vi "Updater Install Spartan Service.vi"(8 "error in (no error)":errorcluster, 11 "Spartan Install Path":path) -> (0 "error out":errorcluster)   [LabVIEW 2011]
uses:
  <vilib>/registry/registry.llb/Write Registry Value Simple U32.vi
  <vilib>/registry/registry.llb/Write Registry Value Simple STR.vi
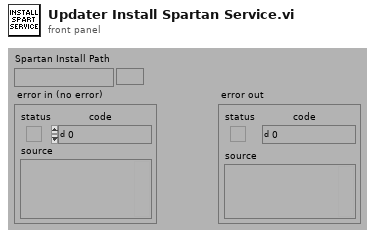
[diagram p1: front panel]
types:
  T1 = typedef "Registry refnum.ctl" = refnum<k1>
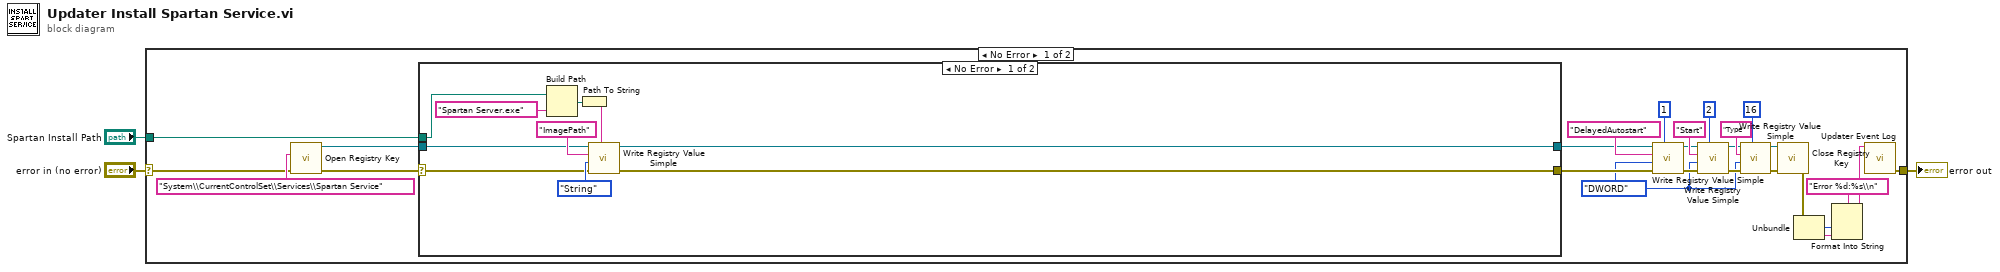
[diagram p0: block diagram]
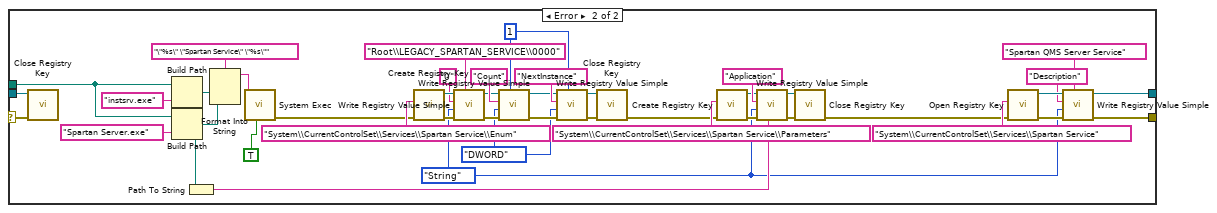
[diagram p2: hidden frame]
diagram:
  n1 = case shown="No Error" "error in (no error)" {
    selector: "error in (no error)" -> [w27 w83]
    tunnel: [w15 w83] -> w3
    tunnel: "Spartan Install Path" -> [w29 _]
    frame No Error {
      w4 = enum16{"String", "Binary", "DWORD"}."DWORD" ("simple data type")
      n2 = call <vilib>:"Open Registry Key.vi"("error in (no error)"=w27, "subkey"="System\\CurrentControlSet\\Services\\Spartan Service") -> ("error out"=w26:errorcluster, "refnum out"=w25:T1)  [unwired: 8 in]
      n3 = case shown="No Error" w26 {
        selector: w26 -> [w37 w46]
        tunnel: [w34 w40] -> w10
        tunnel: w29 -> [w33 w76]
        tunnel: w25 -> [w36 w45]
        tunnel: [w35 w41] -> w5
        frame No Error {
          n4 = Build Path(base path=w33, name or relative path="Spartan Server.exe") -> (appended path=w31:path)
          n5 = Path To String(path=w31) -> (string=w30:string)
          n6 = call-poly <vilib>:"Write Registry Value Simple.vi"("String/Binary data"=w30, "error in (no error)"=w37, "simple data type"=enum16{"String", "Binary", "DWORD"}."String", "value"="ImagePath" ("format string"), "refnum"=w36) -> ("error out"=w34:errorcluster, "refnum out"=w35:T1)  [unwired: 3 in]
        }
        frame Error {
          w44 = enum16{"String", "Binary", "DWORD"}."String" ("simple data type")
          w61 = enum16{"String", "Binary", "DWORD"}."DWORD" ("simple data type")
          w68 = 1
          n7 = call <vilib>:"Close Registry Key.vi"("error in (no error)"=w46, "refnum"=w45) -> ()  [unwired: 5 in, 1 out]
          n8 = Build Path(base path=w76, name or relative path="instsrv.exe") -> (appended path=w80:path)
          n9 = Build Path(base path=w76, name or relative path="Spartan Server.exe") -> (appended path=w55:path)
          n10 = Path To String(path=w55) -> (string=w52:string)
          n11 = Format Into String(format string="\"%s\" \"Spartan Service\" \"%s\"", w80, w55) -> (resulting string=w78:string)  [unwired: 2 in, 1 out]
          n12 = call <vilib>:"System Exec.vi"("run minimized? (F)"=TRUE, "command line"=w78) -> ("error out"=w42:errorcluster)  [unwired: 6 in, 3 out]
          n13 = call <vilib>:"Create Registry Key.vi"("error in (no error)"=w42, "subkey"="System\\CurrentControlSet\\Services\\Spartan Service\\Enum") -> ("error out"=w74:errorcluster, "refnum out"=w73:T1)  [unwired: 7 in, 1 out]
          n14 = call-poly <vilib>:"Write Registry Value Simple.vi"("String/Binary data"="Root\\LEGACY_SPARTAN_SERVICE\\0000" ("format string"), "error in (no error)"=w74, "simple data type"=w44, "value"="0" ("format string"), "refnum"=w73) -> ("error out"=w66:errorcluster, "refnum out"=w67:T1)  [unwired: 3 in]
          n15 = call-poly <vilib>:"Write Registry Value Simple.vi"("DWORD data"=w68, "error in (no error)"=w66, "simple data type"=w61, "value"="Count" ("format string"), "refnum"=w67) -> ("error out"=w65:errorcluster, "refnum out"=w64:T1)  [unwired: 3 in]
          n16 = call-poly <vilib>:"Write Registry Value Simple.vi"("DWORD data"=w68, "error in (no error)"=w65, "simple data type"=w61, "value"="NextInstance" ("format string"), "refnum"=w64) -> ("error out"=w62:errorcluster, "refnum out"=w63:T1)  [unwired: 3 in]
          n17 = call <vilib>:"Close Registry Key.vi"("error in (no error)"=w62, "refnum"=w63) -> ("error out"=w56:errorcluster)  [unwired: 5 in]
          n18 = call <vilib>:"Create Registry Key.vi"("error in (no error)"=w56, "subkey"="System\\CurrentControlSet\\Services\\Spartan Service\\Parameters") -> ("error out"=w58:errorcluster, "refnum out"=w59:T1)  [unwired: 7 in, 1 out]
          n19 = call-poly <vilib>:"Write Registry Value Simple.vi"("String/Binary data"=w52, "error in (no error)"=w58, "simple data type"=w44, "value"="Application" ("format string"), "refnum"=w59) -> ("error out"=w54:errorcluster, "refnum out"=w53:T1)  [unwired: 3 in]
          n20 = call <vilib>:"Close Registry Key.vi"("error in (no error)"=w54, "refnum"=w53) -> ("error out"=w43:errorcluster)  [unwired: 5 in]
          n21 = call <vilib>:"Open Registry Key.vi"("error in (no error)"=w43, "subkey"="System\\CurrentControlSet\\Services\\Spartan Service") -> ("error out"=w49:errorcluster, "refnum out"=w50:T1)  [unwired: 8 in]
          n22 = call-poly <vilib>:"Write Registry Value Simple.vi"("String/Binary data"="Spartan QMS Server Service" ("format string"), "error in (no error)"=w49, "simple data type"=w44, "value"="Description" ("format string"), "refnum"=w50) -> ("error out"=w40:errorcluster, "refnum out"=w41:T1)  [unwired: 3 in]
        }
      }
      n23 = call-poly <vilib>:"Write Registry Value Simple.vi"("DWORD data"=1, "error in (no error)"=w10, "simple data type"=w4, "value"="DelayedAutostart" ("format string"), "refnum"=w5) -> ("error out"=w9:errorcluster, "refnum out"=w6:T1)  [unwired: 3 in]
      n24 = call-poly <vilib>:"Write Registry Value Simple.vi"("DWORD data"=2, "error in (no error)"=w9, "simple data type"=w4, "value"="Start" ("format string"), "refnum"=w6) -> ("error out"=w8:errorcluster, "refnum out"=w7:T1)  [unwired: 3 in]
      n25 = call-poly <vilib>:"Write Registry Value Simple.vi"("DWORD data"=16, "error in (no error)"=w8, "simple data type"=w4, "value"="Type" ("format string"), "refnum"=w7) -> ("error out"=w22:errorcluster, "refnum out"=w23:T1)  [unwired: 3 in]
      n26 = call <vilib>:"Close Registry Key.vi"("error in (no error)"=w22, "refnum"=w23) -> ("error out"=w16:errorcluster)  [unwired: 5 in]
      n27 = Unbundle(w16) -> ("code"=w19:i32, "source"=w18:string)  [unwired: 1 out]
      n28 = Format Into String(format string="Error %d:%s\\n" ("pattern"), w19, w18) -> (resulting string=w17:string)  [unwired: 2 in, 1 out]
      n29 = call "Updater Event Log.vi"("Log Entry"=w17) -> ("error out"=w15:errorcluster)  [unwired: 1 in, 9 out]
    }
    frame Error {
    }
  }
  "error out" <- w3
